vi "AddChild.vi"(8 "error in (no error)":errorcluster, 10 "Object":refnum<class "Pgui_Obj.lvclass">, 11 "reference in":refnum<class "HGrid.lvclass">) -> (0 "error out":errorcluster, 3 "reference out":refnum<class "HGrid.lvclass">)   [LabVIEW 2019, in "HGrid.lvclass"]
uses:
  HGrid.lvclass
  C:/Users/Taylor.Hillegeist/OneDrive - Ultra/LabVIEW/Pgui2/Pgui_Obj_class/Pgui_Obj.lvclass
  Pgui_Obj_class/Pgui_Obj.lvclass
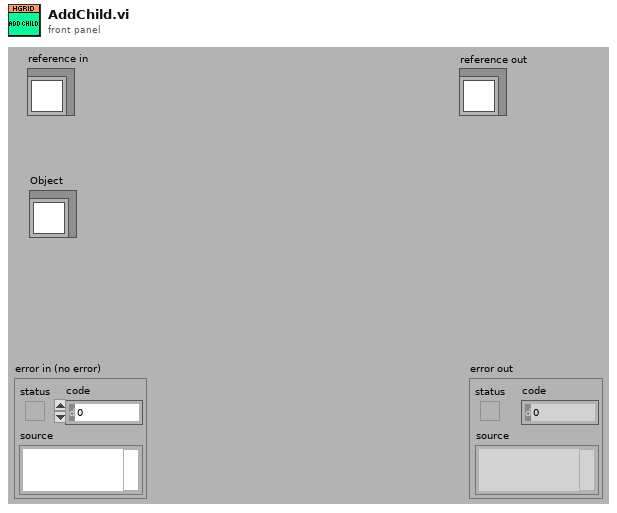
[diagram p1: front panel]
types:
  T1 = typedef "Pgui_Obj.lvclass/ObjectAttributes.ctl" = cluster{"Children":refnum<class "Pgui_Obj.lvclass">[], "Draw Instr":picture, "Params":cluster{"left":i16, "top":i16, "right":i16, "bottom":i16}, "Parent_Pgui_Obj":refnum<class "Pgui_Obj.lvclass">, "MouseOver":bool}
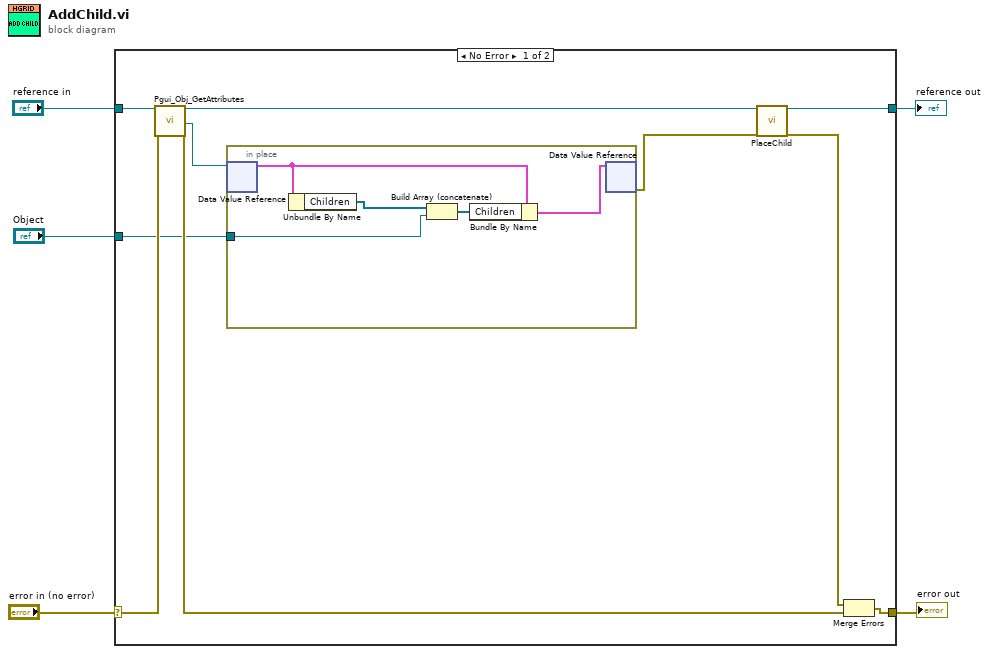
[diagram p0: block diagram]
diagram:
  n1 = case shown="No Error" "error in (no error)" {
    selector: "error in (no error)" -> [w15 w22]
    tunnel: [w8 w22] -> w4
    tunnel: [w6 w21] -> w2
    tunnel: "reference in" -> [w13 w21]
    tunnel: "Object" -> [w11 _]
    frame No Error {
      n2 = call "Pgui_Obj_GetAttributes.vi"("reference in"=w13, "error in (no error)"=w15) -> ("reference out"=w10:refnum<class "HGrid.lvclass">, "DataRef"=w12:refnum<data-value>, "error out"=w14:errorcluster)  [unwired: 14 in, 1 out]
      n3 = in-place {
        in-place-border: w11 -> [w18]
        n4 = in-place-dvr #1(w12) -> (w19:T1)  [unwired: 1 out]
        n5 = Unbundle By Name(w19) -> ("Children"=w17:refnum<class "Pgui_Obj.lvclass">[])
        n6 = Build Array (concatenate)(w17, w18) -> (w16:refnum<class "Pgui_Obj.lvclass">[])
        n7 = Bundle By Name(cluster=w19, "Children"=w16) -> (w20:T1)
        n8 = in-place-dvr #1(w20) -> (w9:errorcluster)  [unwired: 1 out]
      }
      n9 = call-dynamic "PlaceChild.vi"("reference in"=w10, "error in (no error)"=w9) -> ("reference out"=w6:refnum<class "HGrid.lvclass">, "error out"=w7:errorcluster)  [unwired: 16 in]
      n10 = Merge Errors(w7, w14) -> (w8:errorcluster)
    }
    frame Error {
    }
  }
  "error out" <- w4
  "reference out" <- w2
